vi "Read IsStopped.vi"(8 "error in (no error)":errorcluster, 11 "ExperimentService in":refnum<class "ExperimentService.lvclass">) -> (0 "error out":errorcluster, 2 "IsStopped":bool, 3 "ExperimentService out":refnum<class "ExperimentService.lvclass">)   [LabVIEW 2014, in "ExperimentService.lvclass"]
uses:
  ExperimentService.lvclass
  ExperimentService.lvclass/ExperimentService.ctl
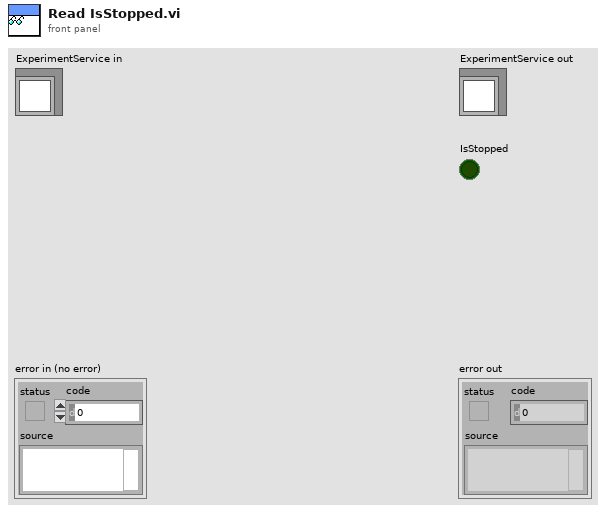
[diagram p1: front panel]
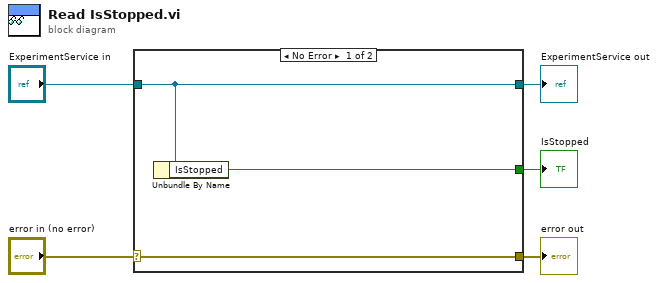
[diagram p0: block diagram]
diagram:
  n1 = case shown="No Error" "error in (no error)" {
    selector: "error in (no error)" -> [w8 w9]
    tunnel: [w8 w9] -> w4
    tunnel: [w7 w10] -> w2
    tunnel: "ExperimentService in" -> [w7 w10]
    tunnel: [w6 _] -> w1
    frame No Error {
      n2 = Unbundle By Name(w7) -> ("IsStopped"=w6:bool)
    }
    frame Error {
    }
  }
  "error out" <- w4
  "ExperimentService out" <- w2
  "IsStopped" <- w1
